vi "LDT Test Program.vi"() -> ()   [LabVIEW 2024, in "LDT Telescope.lvclass"]
uses:
  LDT Telescope.lvclass
  Telescope cluster Status.ctl
  typedefs/CC cluster RA and DEC.ctl
  Telescope enum Status.ctl
  typedefs/CC cluster Object.ctl
  typedefs/CC cluster sidereal rate.ctl
  typedefs/cc cluster muRA muDEC.ctl
  CC cluster Telescope Offsets.ctl
  Telescope cluster Equinox.ctl
  Telescope cluster Parallax.ctl
  Telescope cluster Rotator.ctl
  Telesope ring Frame.ctl
  Telescope.lvclass
panel:
  in  "Object":T1
  in  "Send":bool
  out "error out":errorcluster
  in  "Stop Button":bool
  out "Raw Response":string
  out "Telescope Status":T10
  out "Connect Message":string
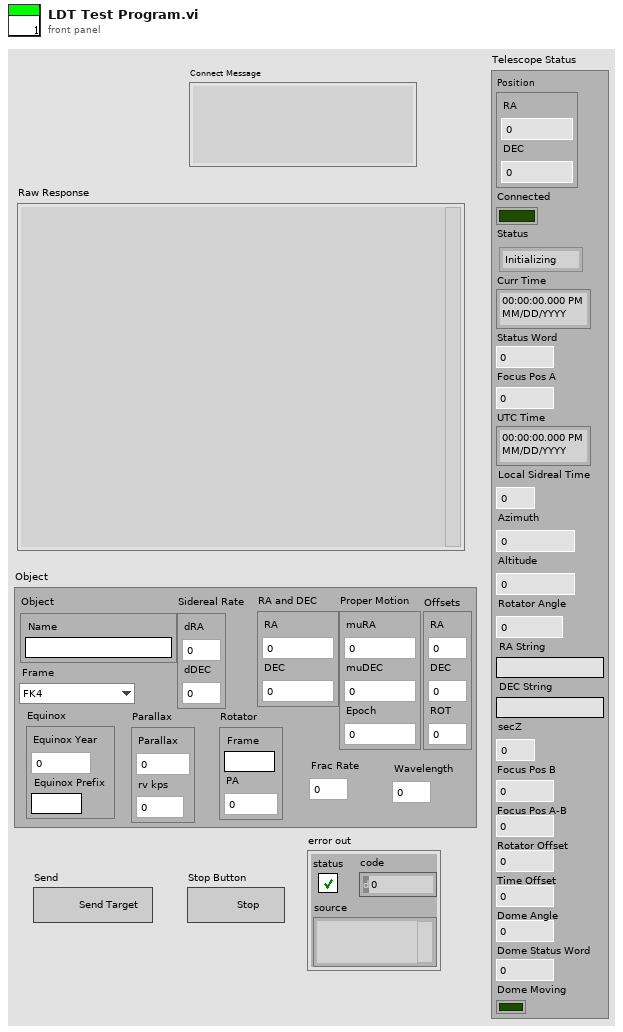
[diagram p1: front panel]
types:
  T1 = typedef "CC cluster Object.ctl" = cluster{"Object":cluster{"Name":string}, "Sidereal Rate":T2, "RA and DEC":T3, "Proper Motion":T4, "Offsets":T5, "Equinox":T6, "Parallax":T7, "Rotator":T8, "Frame":T9, "Frac Rate":dbl, "Wavelength":dbl}
  T2 = typedef "CC cluster sidereal rate.ctl" = cluster{"dRA":dbl, "dDEC":dbl}
  T3 = typedef "CC cluster RA and DEC.ctl" = cluster{"RA":dbl, "DEC":dbl}
  T4 = typedef "cc cluster muRA muDEC.ctl" = cluster{"muRA":dbl, "muDEC":dbl, "Epoch":dbl}
  T5 = typedef "CC cluster Telescope Offsets.ctl" = cluster{"RA":dbl, "DEC":dbl, "ROT":dbl}
  T6 = typedef "Telescope cluster Equinox.ctl" = cluster{"Equinox Year":i32, "Equinox Prefix":string}
  T7 = typedef "Telescope cluster Parallax.ctl" = cluster{"Parallax":dbl, "rv kps":dbl}
  T8 = typedef "Telescope cluster Rotator.ctl" = cluster{"Frame":string, "PA":dbl}
  T9 = typedef "Telesope ring Frame.ctl" = enum16{"FK4", "FK5", "APPT", "GAPPT", "AZEL"}
  T10 = typedef "Telescope.lvclass/Telescope cluster Status.ctl" = cluster{"Position":T3, "Connected":bool, "Status":T11, "Curr Time":timestamp, "Status Word":u32, "Focus Pos A":dbl, "UTC Time":timestamp, "Local Sidreal Time":dbl, "Azimuth":dbl, "Altitude":dbl, "Rotator Angle":dbl, "RA String":string, "DEC String":string, "secZ":dbl, "Focus Pos B":dbl, "Focus Pos A-B":dbl, "Rotator Offset":dbl, "Time Offset":dbl, "Dome Angle":dbl, "Dome Status Word":u32, "Dome Moving":bool}
  T11 = typedef "Telescope.lvclass/Telescope enum Status.ctl" = enum16{"Initializing", "Ready", "Moving", "Focusing", "Error"}
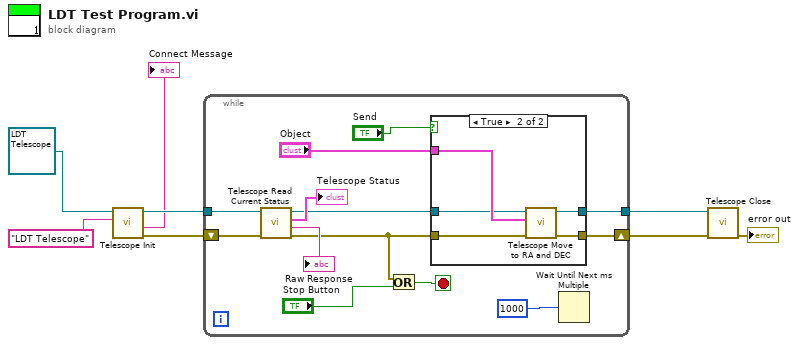
[diagram p0: block diagram]
diagram:
  n1 = call-dynamic "Telescope Init.vi"("Name"="LDT Telescope", "LDT Telescope in"=refnum<class "LDT Telescope.lvclass"> refnum ("LDT Telescope.lvclass")) -> ("error out"=w4:errorcluster, "Connect Message"=→"Connect Message":string, "LDT Telescope out"=w6:refnum<class "LDT Telescope.lvclass">)  [unwired: 6 in, 1 out]
  n2 = while {
    tunnel: w6 -> [w21]
    shift-right: [w11] -> w3
    shift-left: w4 -> [w20]
    tunnel: [w9] -> w2
    stop <- w17 stop-if-true
    n3 = call-dynamic "Telescope Read Current Status.vi"("error in (no error)"=w20, "LDT Telescope in"=w21) -> ("error out"=w12:errorcluster, "Raw Response"=→"Raw Response":string, "Telescope Status"=→"Telescope Status":T10, "LDT Telescope out"=w10:refnum<class "LDT Telescope.lvclass">)  [unwired: 5 in, 1 out]
    n4 = Or(x=w12, y="Stop Button") -> (x .or. y?=w17:bool)
    n5 = case shown="True" "Send" {
      tunnel: "Object" -> [_ w28]
      tunnel: w12 -> [w22 w27]
      tunnel: [w22 w26] -> w11
      tunnel: w10 -> [w23 w25]
      tunnel: [w23 w24] -> w9
      frame False {
      }
      frame True {
        n6 = call-dynamic "Telescope Move to RA and DEC.vi"("error in (no error)"=w27, "Object out"=w28, "LDT Telescope in"=w25) -> ("error out"=w26:errorcluster, "LDT Telescope out"=w24:refnum<class "LDT Telescope.lvclass">)  [unwired: 7 in]
      }
    }
    n7 = Wait Until Next ms Multiple(millisecond multiple=u32 1000) -> ()  [unwired: 1 out]
  }
  n8 = call-dynamic "Telescope Close.vi"("error in (no error)"=w3, "LDT Telescope in"=w2) -> ("error out"=→"error out":errorcluster)  [unwired: 8 in, 1 out]
